vi "trace_math_spectra_binaryMath.vi"(0 "reference in":refnum<class "OSA.lvclass">, 1 "spectrum1 trace idx":u32, 2 "spectrum2 trace idx":u32, 5 "error in (no error)":errorcluster) -> (13 "global absorbance trace idx":u32, 14 "reference out":refnum<class "OSA.lvclass">, 19 "error out":errorcluster)   [LabVIEW 2010, in "OSA.lvclass"]
doc: "Performs the math_operand operation on the two spectra. \n\nParameters\n\nspectrum1: this is parameter one to the input and is also the output.\n\nspectrum2: this is parameter two to the input and will not be modified.\n\noperator: The operation to perform, this must be one of the operator_spectrum_... operations as defined in FTSMath.h. \n \nReturnsFTS_SUCCESS if the operation succeeds. FTS_ERROR_RANGE_ERROR if the two spectra are not of the same length FTS_ERROR_PARAMETER_ERROR if the operand is of the wrong type ."
uses:
  OSA.lvclass
  typeDef/acq_dataType.ctl
  FTSLib.dll
panel:
  in  "operator":T1(ring)
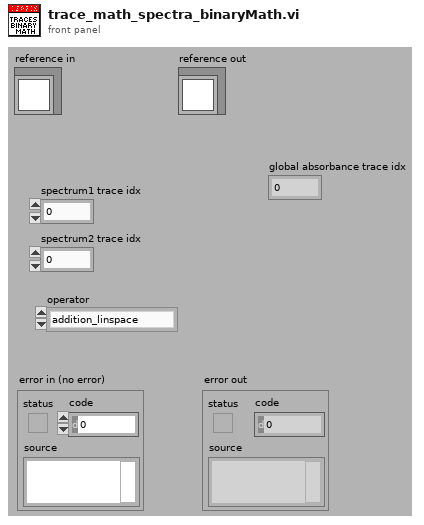
[diagram p1: front panel]
types:
  T1 = enum16{"addition_linspace", "addition_logspace", "subtraction_linspace", "subtraction_logspace", "multiplication", "division"}
  T2 = typedef "OSA.lvclass/acq_dataType.ctl" = enum16{"none", "interferogram", "spectrum"}
  T3 = typedef "OSA.lvclass/ObjectAttributes.ctl" = cluster{"Stop":bool, "dataType":T2, "spectrometerIdx":u16, "buffer size interferogram":i32, "interferogram":cluster{"new":bool, "plot_x_ min":sgl, "plot_x_max":sgl, "plot_y_min":sgl, "plot_y_max":sgl, "Graph Intrfrgrm":T4, "timeStamp":u32, "signal (%)":dbl, "traces":cluster{"idx":u32, "broadBand":bool, "monoChromatic":bool, "peakToPeakSignal":dbl, "peakToPeakPos":dbl}[], "traces idx last":i32}, "spectrum":cluster{"new":bool, "plot_x_min":sgl, "plot_x_max":sgl, "plot_unit_x":T5, "plot_unit_y":T6, "plot_y_min":sgl, "plot_y_max":sgl, "Graph Spectrum":T4, "timeStamp":u32, "X_VAL_OPTIONS":enum16{"MIN_MAX", "ARRAY"}, "traces":cluster{"idx":u32}[], "traces idx last":i32}, "Thorlabs_OSA_64.lvclass:queue_action.ctlqueue ref":refnum<queue>, "action":T7, "plot zoom step":dbl, "buffer semaphore":T8, "acq stopped":bool, "dataType active":T2, "temperature (degr C)":sgl, "pressure (hPa)":sgl, "rel humidity (%)":sgl, "settings":cluster{"resolution":u16, "sensitivity":u16, "Average":bool, "average nr":u32, "apodisation":T9, "acq delay (ms)":u32, "airMesure":T10, "wmtr on":bool, "intfgrm_smooth_width":u16, "intfgrm_smooth_nrOfPasses":u16, "intfgrm_smooth":T11, "phaseCorrection":T12, "zeroFill":u8, "spectr_smooth":T11, "spectr_smooth_width":u16, "spectr_smooth_nrOfPasses":u16, "resolution (/cm)":sgl, "REF wavelength, (nm)":dbl, "gain_idx":u16, "gainAuto":bool, "gain_relative":dbl, "PD sensitivity mode":T13, "PD senseMode implemented":bool, "SensorTemperature implemented":bool, "SensorPressure implemented":bool, "SensorHumidity implemented":bool, "attenuationAuto":bool, "attenuationOnOff":bool, "attenuationAvailable":bool, "offsetAvailable":bool, "offset":i32, "offset max":u16}, "peaks position":sgl[], "peaks width":sgl[], "peaks height":sgl[], "peaks max nr":u32, "peaks latest nr":i32, "peaks new":bool, "power":dbl, "power new":bool, "path":string, "wavelength (WNr)":dbl, "wavelength new":bool, "buffer size spectrum":i32, "status":string, "vi reference":refnum<vi>, "funcPointer":u64, "libraryPointer":u64, "singleAcquisition":bool, "coherenceLength (cm)":dbl, "coherenceLength new":bool, "spectrometer model":string, "spectrometer serial nr":string, "peaks thld left":sgl[], "peaks thld right":sgl[], "coherenceLength error (cm)":dbl, "ADC bits":u16, "peaks position centroid":sgl[], "peaks height centroid":sgl[], "OSA series":T14, "channel index spectrum":u16, "spectrometer rangeLow, (/cm)":dbl, "spectrometer rangeHigh, (/cm)":dbl, "channel index interferogram":u16}
  T4 = typedef "OSA.lvclass/graph_intensity.ctl" = refnum<vi>
  T5 = typedef "OSA.lvclass/spectrum_x_unit.ctl" = enum16{"wavenr/cm", "THz", "eV", "nm_air", "nm_vac"}
  T6 = typedef "OSA.lvclass/y_unit.ctl" = enum16{"ADC counts", "dBm pwr absolute", "dBm pwr density", "mW pwr absolute", "mW pwr density"}
  T7 = typedef "OSA.lvclass/queue_action.ctl" = enum16{"none", "stop", "GUI_plotInterferogram", "GUI_plotSpectrum", "GUI_plotInterferogramRescale", "GUI_plotSpectrumRescale", "GUI_plotInterferogramReset", "GUI_plotSpectrumReset", "GUI_plotInterferogramAutoScaleY", "GUI_plotSpectrumAutoScaleY", "GUI_plotInterferogramZoomOut", "GUI_plotSpectrumZoomOut", "GUI_plotInterferogramPane", "GUI_plotSpectrumPane", "GUI_plotInterferogramZoomMouse", "GUI_plotSpectrumZoomMouse", "GUI_spectrumChannelType", "GUI_channel", "ENVIRONMENT temperature", "ENVIRONMENT pressure", "MODE_resolution set", "MODE_resolution get", "MODE_sensitivity set", "MODE_sensitivity get", "MODE_PDTemperature set", "MODE_PDTemperature get", "REBOOT/RESET firmware", "ACQASYNC_acquireSingleSpectrum", "ACQASYNC_continuous start", "ACQASYNC_continuous stop\n", "ACQASYNC_get last interferogram", "ACQASYNC_get last spectrum", "ACQASYNC_get last waveNr", "ACQOPT_interferogram smoothing set", "ACQOPT_interferogram smoothing get", "ACQOPT_spectrum smoothing set", "ACQOPT_spectrum smoothing get", "ACQOPT_apodisation type set", "ACQOPT_apodisation type get", "ACQOPT_phase correction type set", "ACQOPT_phase correction type get", "ACQOPT_acqIntervall_set", "ACQOPT_acqIntervall_get", "ACQOPT_average spectrum set", "ACQOPT_average spectrum get", "ACQOPT_rolling average set", "ACQOPT_rolling average get", "ACQOPT_zero fill factor set", "ACQOPT_zero fill factor get", "ACQOPT_cycle counting set", "ACQOPT_cycle counting get", "ACQOPT_air measure option set", "ACQOPT_air measure option get", "ACQOPT_gainLevel auto get", "ACQOPT_gainLevel auto set", "ACQOPT_gainLevel get", "ACQOPT_gainLevel set", "ACQOPT_offset set", "ACQOPT_attenuator_auto_set", "ACQOPT_attenuator_set", "ACQOPT_getAll", "INSTRUMENT_PROPERTY_range_WaveNr_min", "INSTRUMENT_PROPERTY_range_WaveNr_max", "INSTRUMENT_PROPERTY_reference_wavelength_cm^-1", "INSTRUMENT_PROPERTY_samplesPerRefPeriod", "INSTRUMENT_PROPERTY_resolution_waveNrPercm", "INSTRUMENT_PROPERTY_availableGainLevels", "INSTRUMENT_PROPERTY_status", "CONVERT", "ANALYSE_POWER", "ANALYSE_PEAKS", "ANALYSE_WAVELENGTH", "ANALYSE_SPECTRUM", "ANALYSE_INTERFEROGRAM", "ANALYSE_COHERENCE_LENGTH", "MATH", "MATH_power", "MATH_peaks", "FILE", "miscellaneous"}
  T8 = typedef "Semaphore RefNum" = refnum<k1>
  T9 = typedef "OSA.lvclass/apodisation.ctl" = enum16{"NONE", "NORTON_BEER_WEAK", "NORTON_BEER_MEDIUM", "NORTON_BEER_STRONG", "TRIANGULAR", "COSINE", "HANN", "HAMMING", "BLACKMANHARRIS3", "BLACKMANHARRIS4", "GAUSSIAN"}
  T10 = typedef "OSA.lvclass/airMeasure.ctl" = enum16{"TEMPERATURE", "PRESSURE"}
  T11 = typedef "OSA20X_misc.lvlib/interferogram_smoothing.ctl" = enum16{"NONE", "BINOMIAL", "SAVITSKY_GOLAY", "FOURIER", "MOVING_AVERAGE", "GAUSSIAN"}
  T12 = typedef "OSA.lvclass/phaseCorrection.ctl" = enum16{"NONE", "MERTZ", "FORMAN", "MERTZ_FILE", "FORMAN_FILE", "FUTURE COMP."}
  T13 = typedef "OSA20X_misc.lvlib/PDTemperatureMode.ctl" = enum16{"cool: better sensitivity/noise floor", "warm: extended wl range"}
  T14 = typedef "OSA.lvclass/OSA_series.ctl" = enum16{"OSA200", "OSA300", "UNKNOWN"}
  T15 = cluster{"idx":u32, "broadBand":bool, "monoChromatic":bool, "peakToPeakSignal":dbl, "peakToPeakPos":dbl}[]
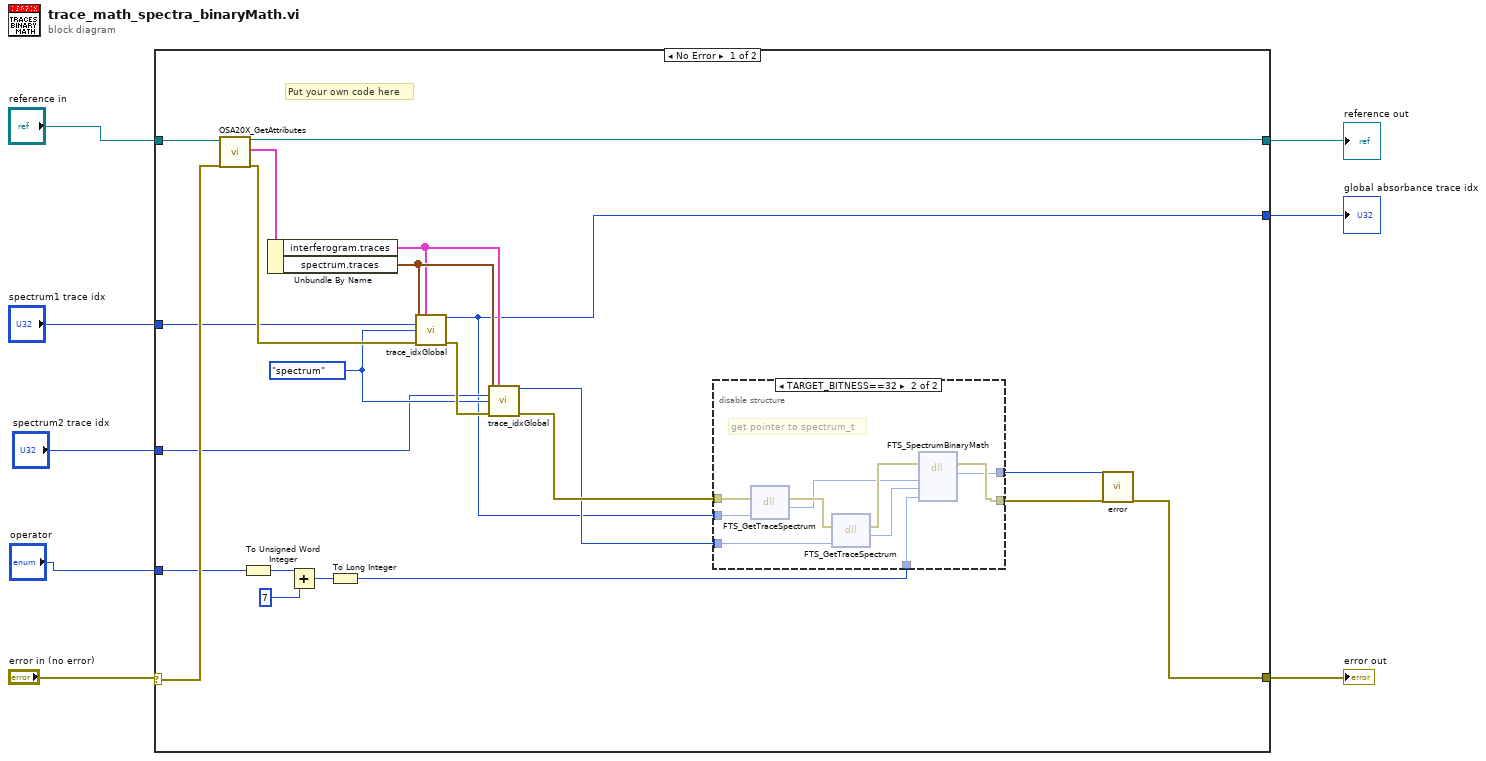
[diagram p0: block diagram]
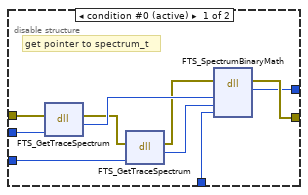
[diagram p2: hidden frame]
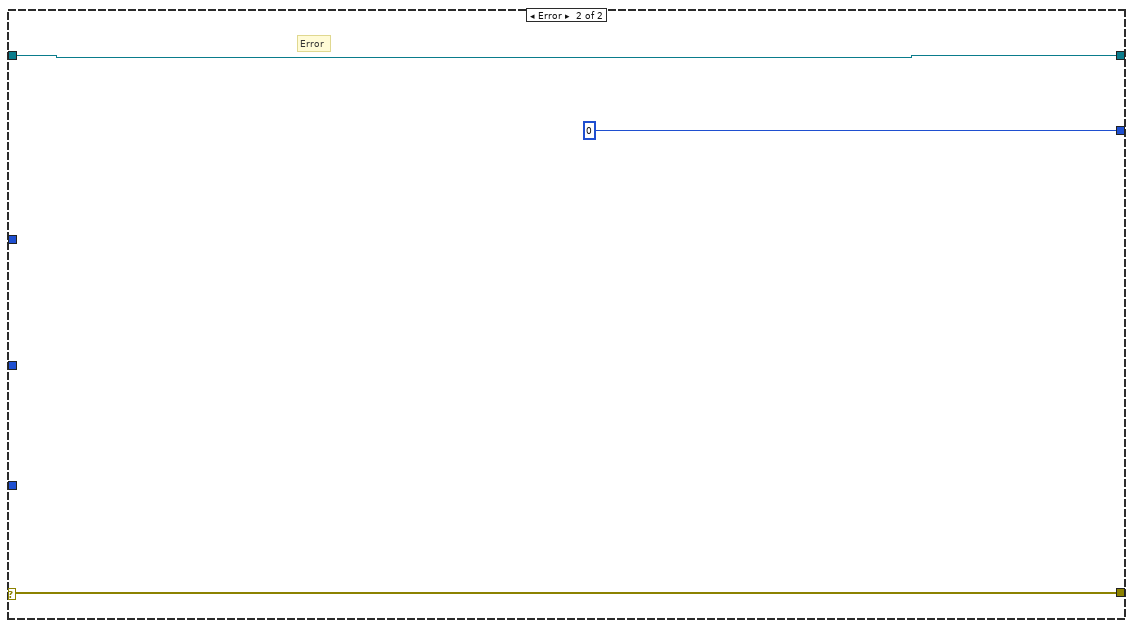
[diagram p3: hidden frame]
diagram:
  n1 = case shown="No Error" "error in (no error)" {
    selector: "error in (no error)" -> [w26 w53]
    tunnel: [w30 w53] -> w8
    tunnel: "reference in" -> [w28 w52]
    tunnel: [w27 w52] -> w3
    tunnel: "spectrum1 trace idx" -> [w24 _]
    tunnel: [w9 u32 0 ("global trace idx")] -> w4
    tunnel: "spectrum2 trace idx" -> [w16 _]
    tunnel: "operator" -> [w15 _]
    frame No Error {
      w17 = acq_dataType."spectrum" ("dataType")
      # "Put your own code here"
      n2 = call "OSA20X_GetAttributes.vi"("reference in"=w28, "error in (no error)"=w26) -> ("reference out"=w27:refnum<class "OSA.lvclass">, "Data"=w29:T3, "error out"=w25:errorcluster)  [unwired: 14 in, 1 out]
      n3 = To Unsigned Word Integer(number=w15) -> (unsigned 16bit integer=w14:u16)
      n4 = Unbundle By Name(w29) -> ("interferogram.traces"=w18:T15, "spectrum.traces"=w19:cluster{"idx":u32}[])
      n5 = Add(x=w14, y=u16 7) -> (x+y=w12:u16)
      n6 = To Long Integer(number=w12) -> (32bit integer=w11:i32)
      n7 = call "trace_idxGlobal.vi"("traces_spectrum"=w19, "traces_interferogram"=w18, "trace idx"=w24, "dataType"=w17, "error in (no error)"=w25) -> ("global trace idx"=w9:u32, "error out"=w21:errorcluster)  [unwired: 9 in]
      n8 = call "trace_idxGlobal.vi"("traces_spectrum"=w19, "traces_interferogram"=w18, "trace idx"=w16, "dataType"=w17, "error in (no error)"=w21) -> ("global trace idx"=w10:u32, "error out"=w20:errorcluster)  [unwired: 9 in]
      n9 = disable-structure shown="TARGET_BITNESS==32" {
        disable-tunnel: w9 -> [w40 w48]
        disable-tunnel: w20 -> [w38 w49]
        disable-tunnel: [w37 w45] -> w23
        disable-tunnel: [w36 w41] -> w22
        disable-tunnel: w10 -> [w33 w47]
        disable-tunnel: w11 -> [w31 w42]
        frame condition #0 (active) {
          # "get pointer to spectrum_t"
          n10 = dll-call lib="FTSLib.dll" fn="FTS_GetTraceSpectrum"(error in=w38, "traceIdx"=w40) -> (error out=w35:errorcluster, "spectrum_t_pointer"=w39:u64)  [unwired: 3 in, 1 out]
          n11 = dll-call lib="FTSLib.dll" fn="FTS_GetTraceSpectrum"(error in=w35, "traceIdx"=w33) -> (error out=w34:errorcluster, "spectrum_t_pointer"=w32:u64)  [unwired: 3 in, 1 out]
          n12 = dll-call lib="FTSLib.dll" fn="FTS_SpectrumBinaryMath"(error in=w34, "spectrum_t_pointer"=w39, "spectrum_t_pointer"=w32, "operator"=w31) -> (error out=w37:errorcluster, "returnVal"=w36:i32)  [unwired: 5 in, 1 out]
        }
        frame condition #1 {
          # "get pointer to spectrum_t"
          n13 = dll-call lib="FTSLib.dll" fn="FTS_GetTraceSpectrum"(error in=w49, "traceIdx"=w48) -> (error out=w50:errorcluster, "spectrum_t_pointer"=w44:u32)  [unwired: 3 in, 1 out]
          n14 = dll-call lib="FTSLib.dll" fn="FTS_GetTraceSpectrum"(error in=w50, "traceIdx"=w47) -> (error out=w46:errorcluster, "spectrum_t_pointer"=w43:u32)  [unwired: 3 in, 1 out]
          n15 = dll-call lib="FTSLib.dll" fn="FTS_SpectrumBinaryMath"(error in=w46, "spectrum_t_pointer"=w44, "spectrum_t_pointer"=w43, "operator"=w42) -> (error out=w45:errorcluster, "returnVal"=w41:i32)  [unwired: 5 in, 1 out]
        }
      }
      n16 = call "error.vi"("result code"=w22, "error in (no error)"=w23) -> ("error out"=w30:errorcluster)  [unwired: 15 in, 2 out]
    }
    frame Error {
      # "Error"
    }
  }
  "error out" <- w8
  "reference out" <- w3
  "global absorbance trace idx" <- w4
